vi "EV Read Serial Atmosphere Editor.vi"(6 "Channel":i32=1, 8 "Calibration in":string, 9 "Hardware in":string, 10 "Setup in":string, 11 "Editor seq info":T1 {"Steps config"."Loop Info"."unit scale" items=["Log", "Lin"]; "Steps config"."Loop Info"."unit dB ref" format="%#_6p"}) -> (1 "Step name out":string="Calibration Default", 2 "Setup out":string, 3 "Sequence channels & curves out":string[](array[string]))   [LabVIEW 2016]
uses:
  custom and Sc run Seq Sub VIs (x64).llb/editor seq info.ctl
  custom and Sc run Seq Sub VIs (x64).llb/Steps config.ctl
  C:/SoundCheck 17/System/Custom VIs/EV.Rotator.RotatorControl.dll
  EV.Rotator.RotatorControl.dll
panel:
  out "Version":string
  in  "Port name":string
  in  "Save as":bool
  in  "save":bool
  in  "revert":bool
  in  "continue loop?":bool
  in  "cancel":bool
  in  "load":bool
  # "This VI will read Temperature, Pressure, and Humidity data into memory list values.\n\nEnter the COM port which is connected to the device."
  # "Reminder:  You must edit this custom step from\nwithin a sequence for it to remember your settings."
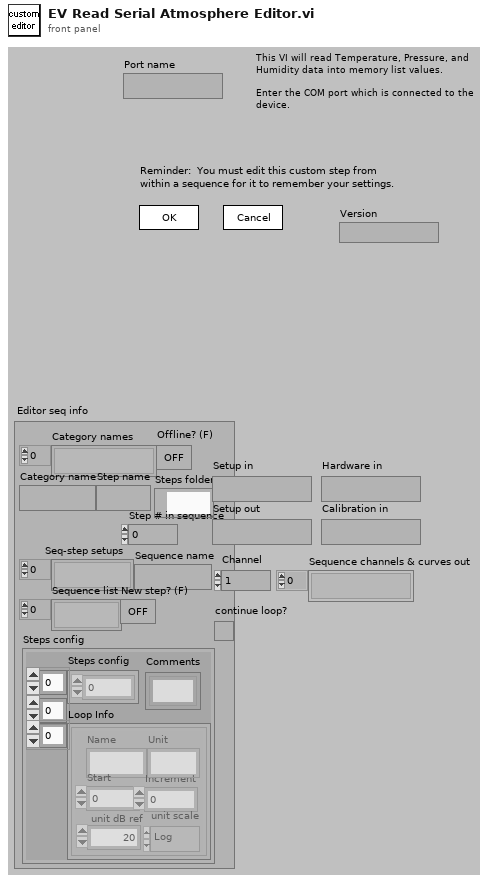
[diagram p1: front panel]
types:
  T1 = typedef "editor seq info.ctl" = cluster{"Category names":string[], "Category name":string, "Step name":string, "Step # in sequence":i32, "Seq-step setups":string[], "Sequence name":string, "Sequence list":string[], "New step? (F)":bool, "Steps config":T2, "Offline? (F)":bool, "Steps folder":path}
  T2 = typedef "Steps config.ctl" = cluster{"Steps config":i32[][], "Loop Info":cluster{"Name":string, "Start":dbl, "Increment":dbl, "Unit":string, "unit dB ref":dbl, "unit scale":u16}[], "Comments":string[]}
  T3 = cluster{"load":bool, "revert":bool, bool, "cancel":bool, "Save as":bool, bool, bool}
  T4 = cluster{"load":bool, "revert":bool, "save":bool, "cancel":bool, "Save as":bool, "close panel":bool, "apply":bool}
  T5 = typedef "seq step setup.ctl" = cluster{"Input Signal Channels":i32[], "Output Signal Channels":i32[], "Curves selected":string[][], "Curves generated":string[], "Step setup flat":string, "Trigger Signal Channel":i32, "Curves Generated Assumptions":cluster{"seq-setup in":string, "Relevant subset of mem list Grouping":cluster{T6[]}[]}}
  T6 = typedef "Memory List Grouping.ctl" = cluster{"item name":string, "parent":string, "Open?":bool, "Type":T7}
  T7 = typedef "Memory List Grouping - Item Type.ctl" = enum16{"item", "custom group", "auto group", "protected group"}
  T8 = typedef "data cluster.ctl" = cluster{"Name":string, "Curve":cluster{"x":dbl, "y":dbl, "z":dbl}[], "X data":T9, "Y data":T9, "Z data":T9, "X axis":u16, "Y axis":u16, "Z axis":u16, "X unit":string, "Y unit":string, "Z unit":string, "X dB ref":dbl, "Y dB ref":dbl, "Z dB ref":dbl, "single val":bool, "protected":bool, "display X":bool, "display Y":bool, "display Z":bool, "Plot Settings":cluster{"Color":u32, "Interpolation":u8, "Point Style":u8, "Line Style":u8, "Point Color":u32, "Line Width":u8, "Bar Plot Style":u8, "Fill To":i16}, "Test Info":string}
  T9 = typedef "Axis Unit Type.ctl" = u16
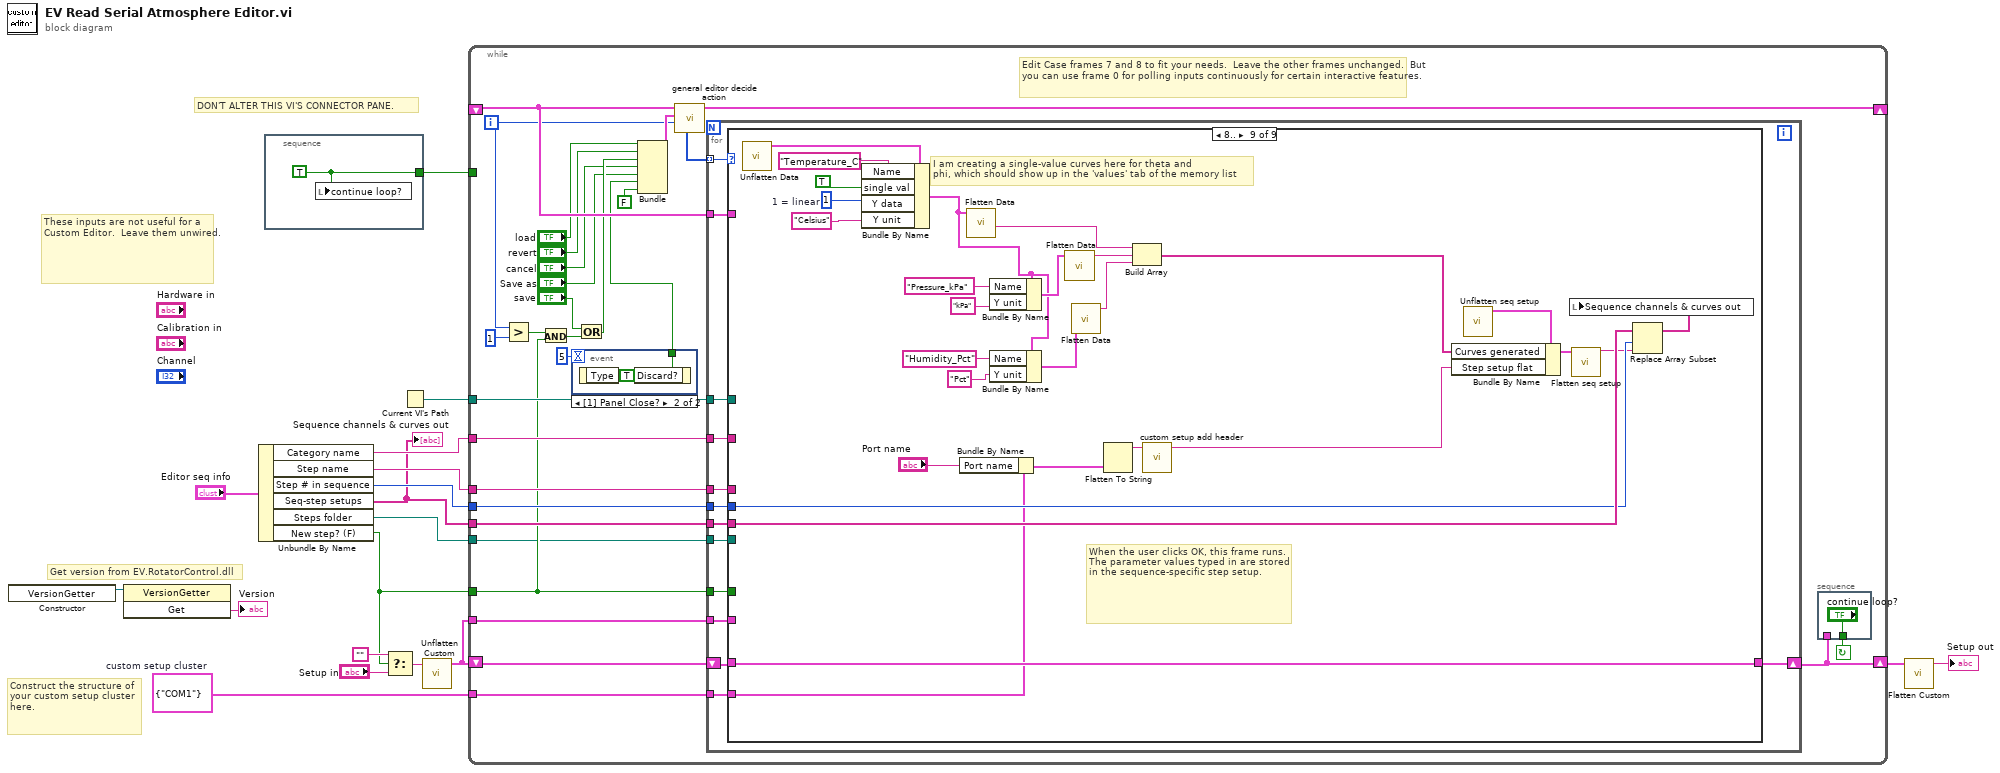
[diagram p0: block diagram]
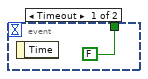
[diagram p2: hidden frame]
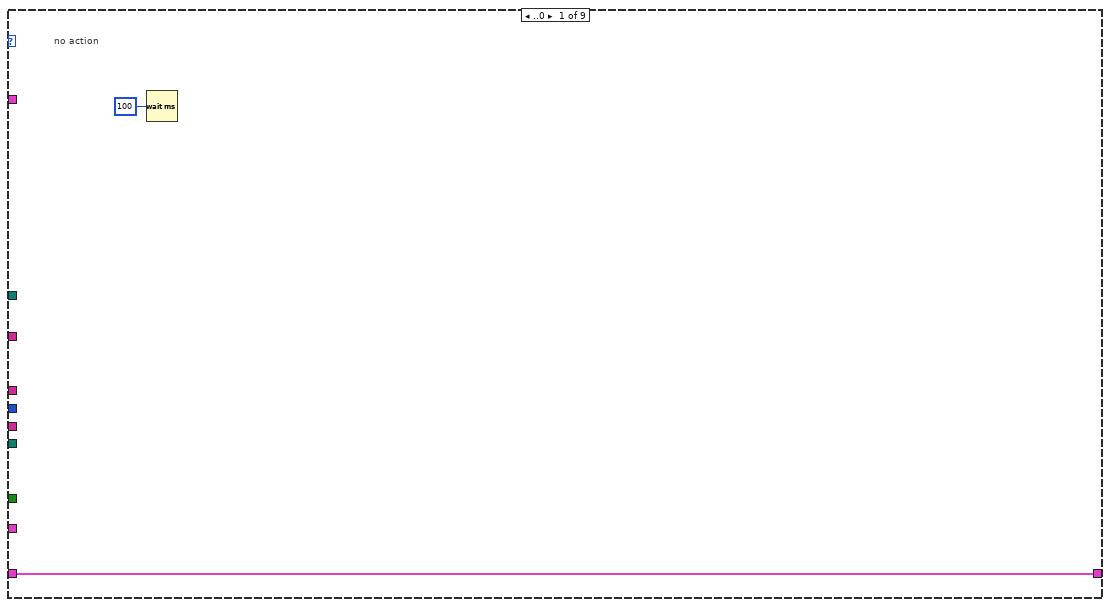
[diagram p3: hidden frame]
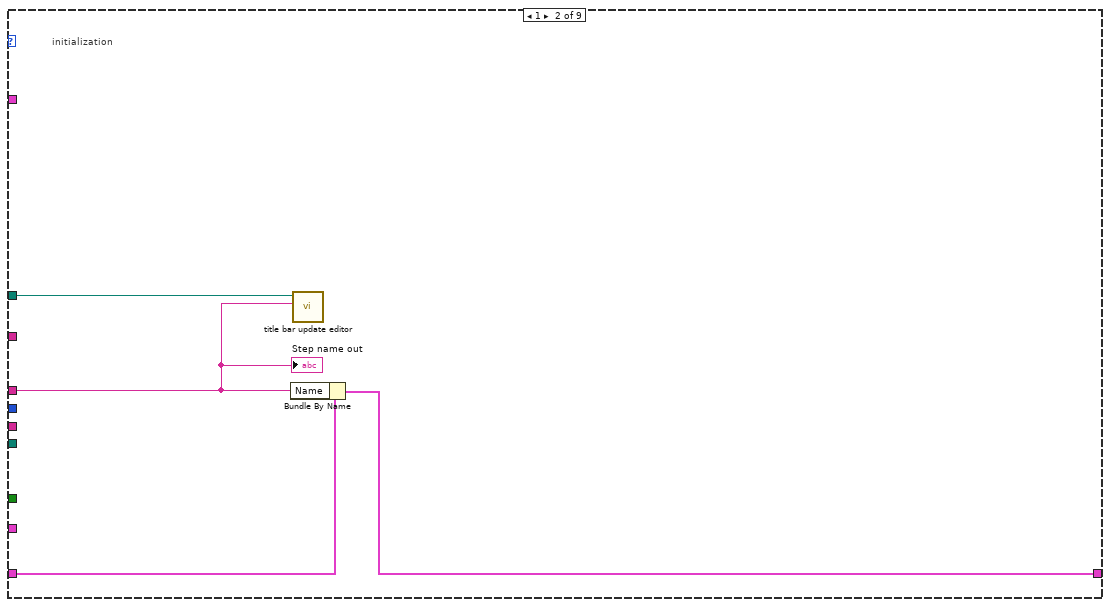
[diagram p4: hidden frame]
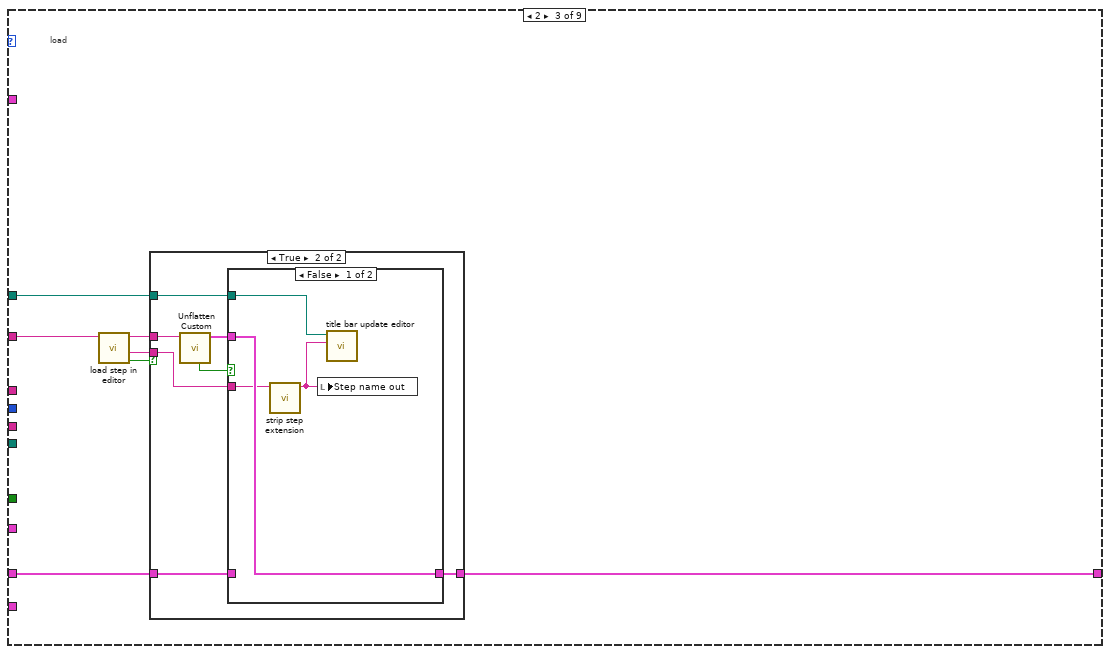
[diagram p5: hidden frame]
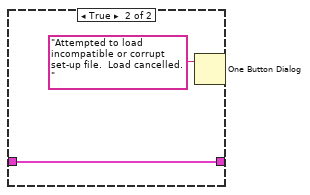
[diagram p7: hidden frame]
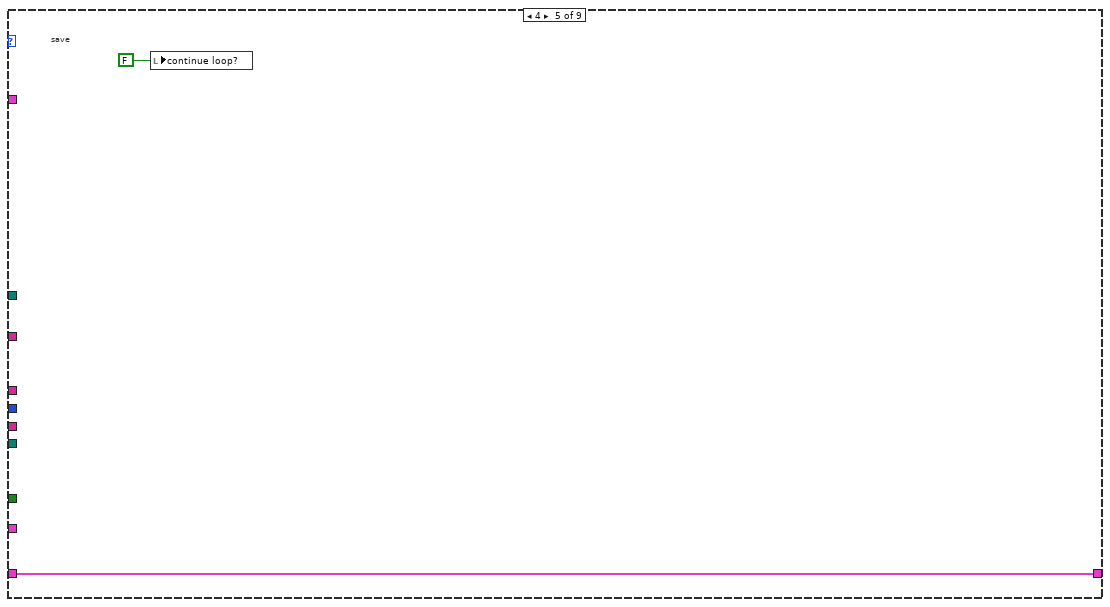
[diagram p9: hidden frame]
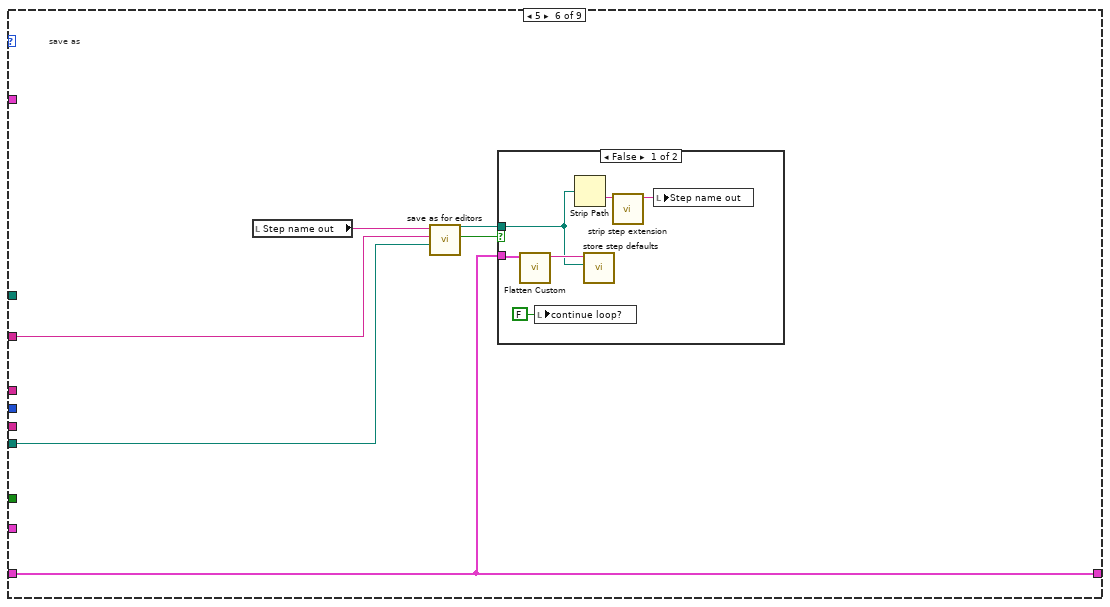
[diagram p10: hidden frame]
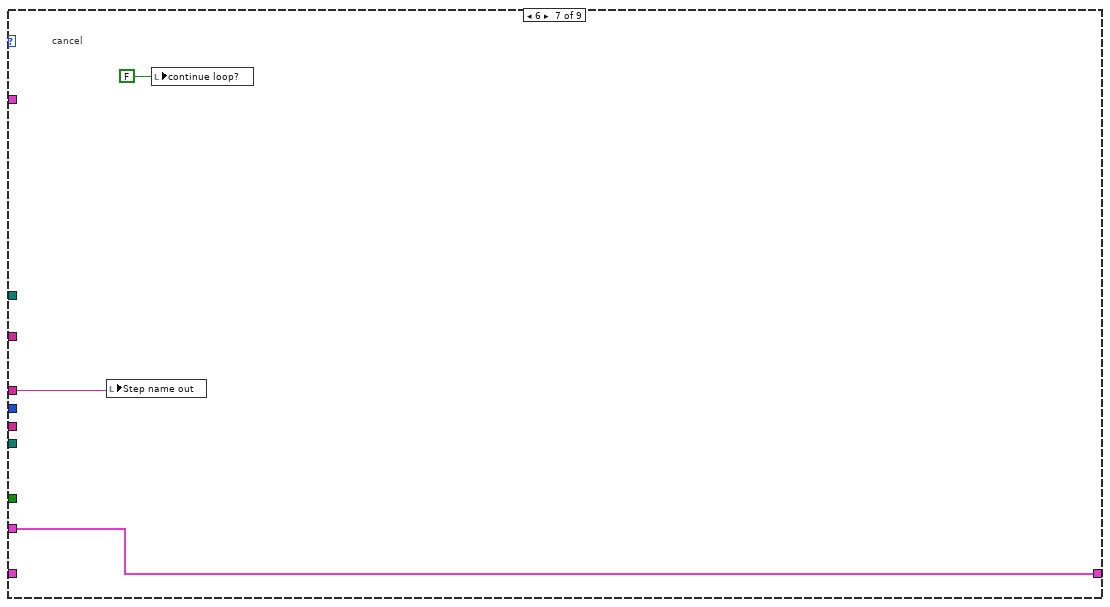
[diagram p12: hidden frame]
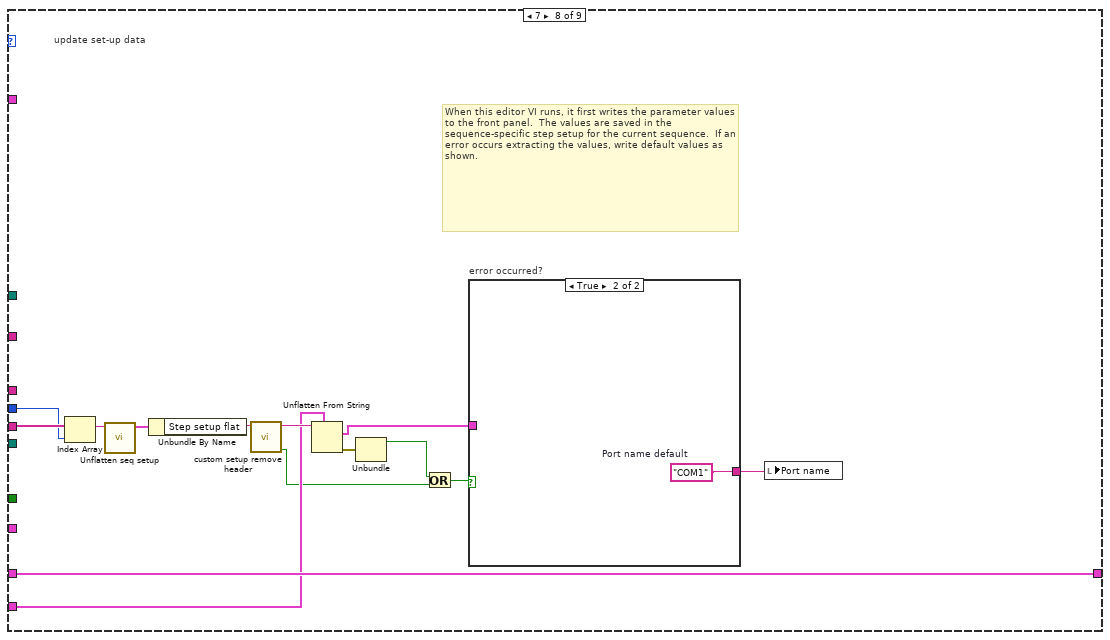
[diagram p13: hidden frame]
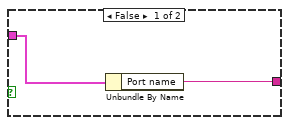
[diagram p14: hidden frame]
diagram:
  w14 = cluster{"Port name":string} {"Port name"="COM1"}  # custom setup cluster
  # "Get version from EV.RotatorControl.dll"
  # "Construct the structure of your custom setup cluster here."
  # "These inputs are not useful for a Custom Editor.  Leave them unwired."
  # "DON'T ALTER THIS VI'S CONNECTOR PANE."
  n1 = constructor class="VersionGetter"() -> (reference out=w1:refnum<k24>)  [unwired: 3 in, 2 out]
  n2 = invoke class="VersionGetter" method="Get"(reference=w1) -> ("Get"=→"Version":string)  [unwired: 2 in, 2 out]
  n3 = Unbundle By Name("Editor seq info") -> ("Category name"=w11:string, "Step name"=w10:string, "Step # in sequence"=w9:i32, "Seq-step setups"=w7:string[], "Steps folder"=w8:path, "New step? (F)"=w4:bool)
  "Sequence channels & curves out" <- w7
  n4 = stacked-sequence {
    tunnel: [w19] -> w12
    frame #0 {
      w19 = TRUE ("continue loop?")
      n5 = local write "continue loop?"(w19) -> ()
    }
  }
  n6 = Select(t="", s=w4, f="Setup in") -> (s? t:f=w15:string)
  n7 = Current VI's Path() -> (path=w13:path)
  n8 = call "Unflatten Custom.vi"("Unflatten Custom"=w15) -> ("Custom"=w3:cluster{"Name":string})  [unwired: 10 out]
  n9 = while {
    tunnel: w14 -> [w29]
    tunnel: w13 -> [w37]
    shift-left: w3 -> [w39]
    shift-right: [w30] -> w5
    tunnel: w3 -> [w41]
    tunnel: w4 -> [w33]
    tunnel: w7 -> [w43]
    tunnel: w9 -> [w44]
    tunnel: w10 -> [w45]
    tunnel: w11 -> [w46]
    shift-left: _ -> [w40]
    shift-right: [w48] -> _
    tunnel: w8 -> [w26]
    tunnel: w12 -> [_]
    i -> [w36]
    stop <- w42 continue-if-true
    # "Edit Case frames 7 and 8 to fit your needs.  Leave the other frames unchanged.  But you can use frame 0 for polling inputs continuously for certain interactive features."
    n10 = Greater?(x=w36, y=1) -> (0:w34:bool)
    n11 = And(x=w34, y=w33) -> (x .and. y?=w32:bool)
    n12 = event shown="[1] Panel Close?" {
      selector: _ -> [_ _]
      dyn-events: _ -> [_ _]
      timeout: 5 -> [_ _]
      tunnel: [FALSE w50] -> w28
      event Timeout {
        n13 = event-data() -> ()  [unwired: 2 out]
      }
      event Panel Close? {
        w50 = TRUE
        n14 = event-data() -> ()  [unwired: 2 out]
        n15 = event-data("Discard?"=w50) -> ()  [unwired: 1 in, 1 out]
      }
    }
    n16 = Or(x="save", y=w32) -> (x .or. y?=w31:bool)
    n17 = Bundle("load"="load", "revert"="revert", w31, "cancel"="cancel", "Save as"="Save as", w28, FALSE) -> (w38:T3)  [unwired: 1 out]
    n18 = call "general editor decide action.vi"("Iteration"=w36, "Polled cluster"=w38, "Old cluster"=w40) -> ("actions array"=w47:i32[], "New cluster"=w48:T4)  [unwired: 1 in, 6 out]
    n19 = for {
      tunnel: w40 -> [w64]
      tunnel: w41 -> [w63]
      tunnel: w33 -> [w62]
      tunnel: w43 -> [w61]
      tunnel: w44 -> [w60]
      tunnel: w45 -> [w59]
      tunnel: w46 -> [w58]
      tunnel: w47 -> [w57] mode=indexing
      shift-right: [w55] -> w30
      shift-left: w39 -> [w56]
      tunnel: w37 -> [w54]
      tunnel: w29 -> [w53]
      tunnel: w26 -> [w52]
      n20 = case shown="8.." w57 {
        tunnel: w58 -> [_ _ w73 _ _ w97 _ _ _]
        tunnel: w59 -> [_ w67 _ _ _ _ w107 _ _]
        tunnel: w60 -> [_ _ _ _ _ _ _ w120 w151]
        tunnel: w61 -> [_ _ _ _ _ _ _ w121 w152]
        tunnel: w62 -> [_ _ _ _ _ _ _ _ _]
        tunnel: w63 -> [_ _ _ w92 _ _ w108 _ _]
        tunnel: [w65 w70 w77 w92 w93 w100 w108 w123 w148] -> w55
        tunnel: w56 -> [w65 w69 w76 _ w93 w100 _ w123 w148]
        tunnel: w64 -> [_ _ _ _ _ _ _ _ _]
        tunnel: w54 -> [_ w68 w71 _ _ _ _ _ _]
        tunnel: w53 -> [_ _ _ _ _ _ _ w116 w145]
        tunnel: w52 -> [_ _ _ _ _ w95 _ _ _]
        frame ..0 {
          # "no action"
          n21 = Wait (ms)(milliseconds to wait=u32 100) -> ()  [unwired: 1 out]
        }
        frame 1 {
          # "initialization"
          n22 = Bundle By Name(cluster=w69, "Name"=w67) -> (w70:cluster{"Name":string})
          n23 = call "title bar update editor.vi"("Step name"=w67, "Editor VI path"=w68) -> ()  [unwired: 10 out]
          "Step name out" <- w67
        }
        frame 2 {
          # "load"
          n24 = call "load step in editor.vi"("Category name"=w73) -> ("Not canceled?"=w74:bool, "New step name (with ext.)"=w72:string, "Flat step set-up"=w75:string)  [unwired: 1 in, 7 out]
          n25 = case shown="True" w74 {
            tunnel: w75 -> [_ w85]
            tunnel: [w78 w83] -> w77
            tunnel: w76 -> [w78 w82]
            tunnel: w72 -> [_ w80]
            tunnel: w71 -> [_ w79]
            frame False {
            }
            frame True {
              n26 = call "Unflatten Custom.vi"("Unflatten Custom"=w85) -> ("Custom"=w81:cluster{"Name":string}, "Error?"=w84:bool)  [unwired: 9 out]
              n27 = case shown="False" w84 {
                tunnel: [w89 w91] -> w83
                tunnel: w82 -> [_ w91]
                tunnel: w81 -> [w89 _]
                tunnel: w80 -> [w88 _]
                tunnel: w79 -> [w87 _]
                frame False {
                  n28 = call "strip step extension.vi"("Step name w/ extension"=w88) -> ("Step name (base)"=w86:string)  [unwired: 1 in, 9 out]
                  n29 = local write "Step name out"(w86) -> ()
                  n30 = call "title bar update editor.vi"("Step name"=w86, "Editor VI path"=w87) -> ()  [unwired: 10 out]
                }
                frame True {
                  n31 = One Button Dialog(message="Attempted to load incompatible or corrupt set-up file.  Load cancelled.") -> ()  [unwired: 2 out]
                }
              }
            }
          }
        }
        frame 3 {
          # "revert"
        }
        frame 4 {
          # "save"
          n32 = local write "continue loop?"(FALSE ("continue loop?")) -> ()
        }
        frame 5 {
          # "save as"
          n33 = local read "Step name out"() -> (w96:string)
          n34 = call "save as for editors.vi"("Steps Folder (gbl if empty)"=w95, "Category name"=w97, "Step name"=w96) -> ("Canceled"=w98:bool, "File path chosen"=w99:path)  [unwired: 3 in, 4 out]
          n35 = case shown="False" w98 {
            tunnel: w99 -> [w102 _]
            tunnel: w100 -> [w105 _]
            frame False {
              n36 = call "Flatten Custom.vi"("Custom"=w105) -> ("Custom flattened"=w106:string)  [unwired: 10 out]
              n37 = local write "continue loop?"(FALSE ("continue loop?")) -> ()
              n38 = Strip Path(path=w102) -> (name=w103:string)  [unwired: 1 out]
              n39 = call "store step defaults.vi"("Set-up file"=w102, "Flat step set-up"=w106) -> ()  [unwired: 4 in, 6 out]
              n40 = call "strip step extension.vi"("Step name w/ extension"=w103) -> ("Step name (base)"=w101:string)  [unwired: 1 in, 9 out]
              n41 = local write "Step name out"(w101) -> ()
            }
            frame True {
            }
          }
        }
        frame 6 {
          # "cancel"
          n42 = local write "Step name out"(w107) -> ()
          n43 = local write "continue loop?"(FALSE ("continue loop?")) -> ()
        }
        frame 7 {
          # "When this editor VI runs, it first writes the parameter values to the front panel.  The values are saved in the sequence-specific step setup for the current sequence.  If an error occurs extracting the values, write default values as shown."
          # "update set-up data"
          n44 = Index Array(array=w121, index=w120) -> (element=w122:string)
          n45 = call "Unflatten seq setup.vi"("Unflatten seq setup"=w122) -> ("Sequence-specific step set-up"=w119:T5)  [unwired: 3 in, 7 out]
          n46 = Unbundle By Name(w119) -> ("Step setup flat"=w118:string)
          n47 = call "custom setup remove header.vi"("Output from 'Step setup flat' of seq-setup structure"=w118) -> ("Error?"=w115:bool, "Flattened custom step setup cluster"=w117:string)  [unwired: 9 out]
          n48 = Unflatten From String(type=w116, binary string=w117) -> (value=w112:cluster{"Port name":string}, error out=w111:errorcluster)  [unwired: 1 in, 3 out]
          n49 = Unbundle(w111) -> ("status"=w114:bool)  [unwired: 2 out]
          n50 = Or(x=w114, y=w115) -> (x .or. y?=w113:bool)
          n51 = case "error occurred?" shown="True" w113 {
            tunnel: w112 -> [w125 _]
            tunnel: [w124 w126] -> w110
            frame False {
              n52 = Unbundle By Name(w125) -> ("Port name"=w124:string)
            }
            frame True {
              w126 = "COM1"  # Port name default
            }
          }
          n53 = local write "Port name"(w110) -> ()
        }
        frame 8.. {
          w139 = u16 1  # 1 = linear
          # "I am creating a single-value curves here for theta and\nphi, which should show up in the 'values' tab of the memory list"
          # "When the user clicks OK, this frame runs.  The parameter values typed in are stored in the sequence-specific step setup."
          n54 = call "Unflatten Data.vi"() -> ("Datum"=w138:T8)  [unwired: 1 in, 10 out]
          n55 = Bundle By Name(cluster=w138, "Name"="Temperature_C", "single val"=TRUE, "Y data"=w139, "Y unit"="Celsius" ("angle in degrees")) -> (w129:T8)
          n56 = Bundle By Name(cluster=w145, "Port name"="Port name") -> (w144:cluster{"Port name":string})
          n57 = call "Flatten Data.vi"("Datum"=w129) -> ("Data flattened"=w141:string)  [unwired: 10 out]
          n58 = Bundle By Name(cluster=w129, "Name"="Pressure_kPa", "Y unit"="kPa" ("X unit")) -> (w134:T8)
          n59 = Bundle By Name(cluster=w129, "Name"="Humidity_Pct", "Y unit"="Pct" ("X unit")) -> (w131:T8)
          n60 = call "Flatten Data.vi"("Datum"=w134) -> ("Data flattened"=w133:string)  [unwired: 10 out]
          n61 = call "Flatten Data.vi"("Datum"=w131) -> ("Data flattened"=w130:string)  [unwired: 10 out]
          n62 = Flatten To String(anything=w144) -> (data string=w146:string)  [unwired: 1 in, 4 out]
          n63 = Build Array(w141, w133, w130) -> (w142:string[])
          n64 = call "custom setup add header.vi"("Flattened custom step setup cluster"=w146) -> ("Input to 'Step setup flat' of seq-setup structure"=w147:string)  [unwired: 1 in, 9 out]
          n65 = call "Unflatten seq setup.vi"() -> ("Sequence-specific step set-up"=w154:T5)  [unwired: 4 in, 7 out]
          n66 = Bundle By Name(cluster=w154, "Curves generated"=w142, "Step setup flat"=w147) -> (w153:T5)
          n67 = call "Flatten seq setup.vi"("Sequence-specific step set-up"=w153) -> ("Seq setup flattened"=w150:string)  [unwired: 10 out]
          n68 = Replace Array Subset(array=w152, new element=w150, index=w151) -> (w149:string[])
          n69 = local write "Sequence channels & curves out"(w149) -> ()
        }
      }
    }
    n70 = stacked-sequence {
      tunnel: ["continue loop?"] -> w42
      tunnel: w30 -> [_]
      frame #0 {
      }
    }
  }
  n71 = call "Flatten Custom.vi"("Custom"=w5) -> ("Custom flattened"=→"Setup out":string)  [unwired: 10 out]
